vi "VI Tree.vi"   [LabVIEW 2012, in "Phidget IR.lvlib"]
doc: "${IR:VITreeHeader}"
uses:
  <instrlib>/Phidgets/Phidget IR/Phidget IR.lvlib
  <instrlib>/Phidgets/Phidget IR/Public/IRStart.vi
  <instrlib>/Phidgets/Phidget IR/Public/IROpen.vi
  <instrlib>/Phidgets/Phidget IR/Public/IRClose.vi
panel:
  # "(c) 2015 Phidgets Inc..  ALL RIGHTS RESERVED."
  # "SEE DIAGRAM\nFOR VI TREE."
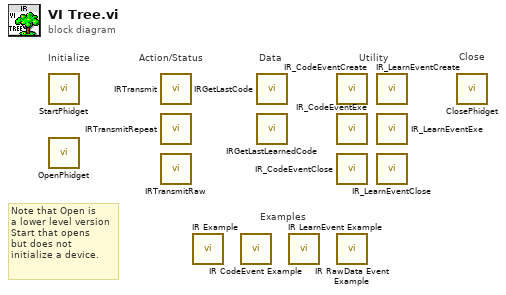
[diagram p0: block diagram]
diagram:
  # "Note that Open is\na lower level version\nStart that opens\nbut does not \ninitialize a device."
  # "Examples"
  # "Utility"
  # "Data"
  # "Action/Status"
  # "Close"
  # "Initialize"
  n1 = call-poly <instrlib>:"StartPhidget.vi"() -> ()  [unwired: 12 in, 4 out]
  n2 = call-poly <instrlib>:"OpenPhidget.vi"() -> ()  [unwired: 8 in, 4 out]
  n3 = call <instrlib>:"IRTransmit.vi"() -> ()  [unwired: 10 in, 2 out]
  n4 = call <instrlib>:"IRTransmitRepeat.vi"() -> ()  [unwired: 9 in, 2 out]
  n5 = call <instrlib>:"IRTransmitRaw.vi"() -> ()  [unwired: 14 in, 2 out]
  n6 = call <instrlib>:"IR Example.vi"() -> ()  [unwired: 12 in]
  n7 = call <instrlib>:"IR CodeEvent Example.vi"() -> ()  [unwired: 12 in]
  n8 = call <instrlib>:"IRGetLastCode.vi"() -> ()  [unwired: 7 in, 4 out]
  n9 = call <instrlib>:"IRGetLastLearnedCode.vi"() -> ()  [unwired: 8 in, 4 out]
  n10 = call <instrlib>:"IR LearnEvent Example.vi"() -> ()  [unwired: 12 in]
  n11 = call <instrlib>:"IR_CodeEventCreate.vi"() -> ()  [unwired: 9 in, 3 out]
  n12 = call <instrlib>:"IR_CodeEventExe.vi"() -> ()  [unwired: 11 in, 9 out]
  n13 = call <instrlib>:"IR_CodeEventClose.vi"() -> ()  [unwired: 10 in, 2 out]
  n14 = call <instrlib>:"IR RawData Event Example.vi"() -> ()  [unwired: 12 in]
  n15 = call <instrlib>:"IR_LearnEventCreate.vi"() -> ()  [unwired: 9 in, 3 out]
  n16 = call <instrlib>:"IR_LearnEventExe.vi"() -> ()  [unwired: 8 in, 8 out]
  n17 = call <instrlib>:"IR_LearnEventClose.vi"() -> ()  [unwired: 10 in, 2 out]
  n18 = call-poly <instrlib>:"ClosePhidget.vi"() -> ()  [unwired: 11 in, 1 out]
